vi "LVClass_Image get Fill Percent.vi"(0 "Image in":refnum<class "Image.lvclass">, 7 "Pixels to Average":u32, 11 "error in (no error)":errorcluster) -> (4 "Image out":refnum<class "Image.lvclass">, 6 "min":u32, 8 "max":u32, 10 "Fill Percent":sgl, 15 "error out":errorcluster)   [LabVIEW 2020, in "Image.lvclass"]
doc: "Image statistics computation.\n\n--------------------------------------------------------------------------------\n\n<B>ImageIn </B> : Image object.\n<B>ImageOut </B> : Image object.\n<B>nb_extreme_pixels </B> : Number of pixels to average for min or max computation.\n<B>min </B> : Average of the nb_extreme_pixels greatest elements.\n<B>max </B> : Average of the nb_extreme_pixels smallest elements.\n<B>fill_percentage </B> : Percentage of saturated pixels.\n<B>ErrorIn </B> : Error\n<B>ErrorOut </B> : Error\n\n--------------------------------------------------------------------------------"
uses:
  Image.lvclass
  Image.lvclass/Image.ctl
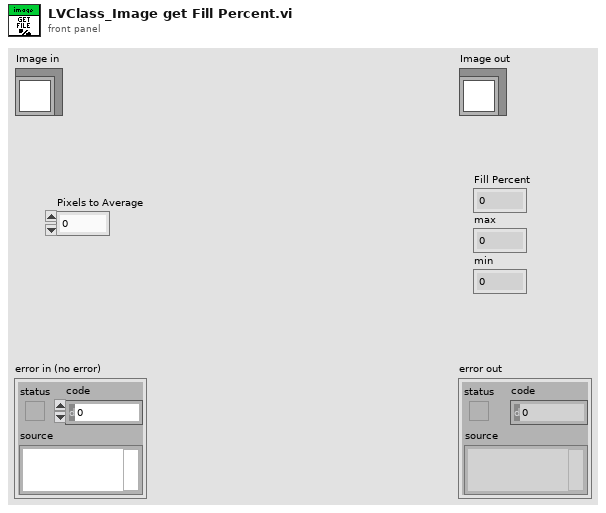
[diagram p1: front panel]
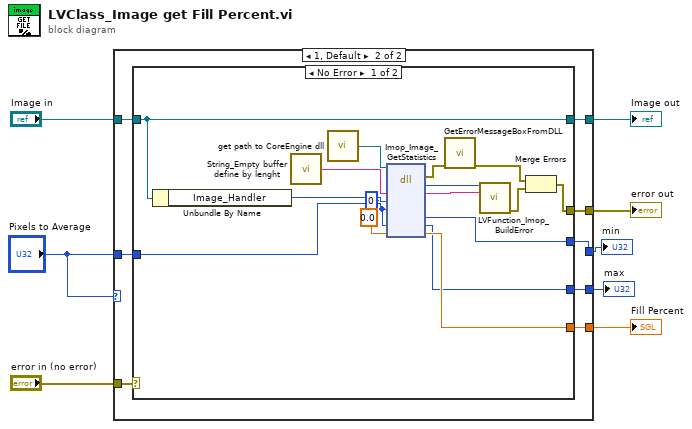
[diagram p0: block diagram]
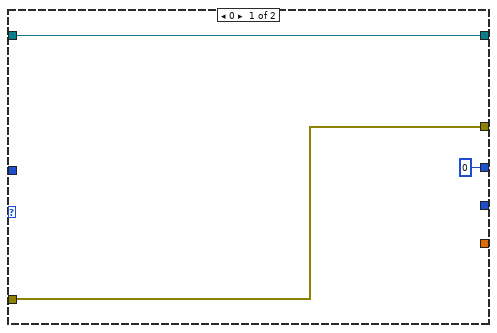
[diagram p2: hidden frame]
diagram:
  n1 = case shown="1, Default" "Pixels to Average" {
    tunnel: "error in (no error)" -> [w10 w19]
    tunnel: [w10 w18] -> w7
    tunnel: "Image in" -> [w11 w17]
    tunnel: [w11 w16] -> w5
    tunnel: [_ w15] -> w4
    tunnel: [u32 0 ("min") w14] -> w3
    tunnel: [_ w13] -> w2
    tunnel: "Pixels to Average" -> [_ w12]
    frame 0 {
    }
    frame 1, Default {
      n2 = case shown="No Error" w19 {
        selector: w19 -> [_ w37]
        tunnel: [w22 w37] -> w18
        tunnel: [w28 w36] -> w16
        tunnel: w17 -> [w28 w36]
        tunnel: [w29 _] -> w15
        tunnel: [w25 _] -> w14
        tunnel: [w24 _] -> w13
        tunnel: w12 -> [w20 _]
        frame No Error {
          n3 = Unbundle By Name(w28) -> ("Image_Handler"=w27:i32)
          n4 = call "String_Empty buffer define by lenght.vi"() -> ("Empty buffer"=w35:string)  [unwired: 1 in]
          n5 = call "get path to CoreEngine dll.vi"() -> ("path to c_interface_vc100.dll"=w32:path)  [unwired: 12 in, 3 out]
          n6 = dll-call lib="D:/soft/HASO_v3/SVN_trunk/ImOpCoreEngine4_LV2011/DLLs/c_interface_vc100.dll" fn="Imop_Image_GetStatistics"(path in=w32, "message"=w35, "Image compat"=w27, "Pixels to Average"=w20, "min"=u32 0, "max"=w20, "Fill_percent"=sgl 0.0 ("Fill Percent")) -> (error out=w31:errorcluster, "return type"=w34:i32, "message"=w33:string, "min"=w25:u32, "max"=w24:u32, "Fill_percent"=w29:sgl)  [unwired: 4 in, 1 out]
          n7 = call "GetErrorMessageBoxFromDLL.vi"("error IN"=w31) -> ("error OUT"=w21:errorcluster)  [unwired: 10 in]
          n8 = call "LVFunction_Imop_BuildError.vi"("code"=w34, "String to Prepend to source (\"\")"=w33) -> ("error out"=w23:errorcluster)  [unwired: 13 in]
          n9 = Merge Errors(w21, w23) -> (w22:errorcluster)
        }
        frame Error {
        }
      }
    }
  }
  "error out" <- w7
  "Image out" <- w5
  "Fill Percent" <- w4
  "min" <- w3
  "max" <- w2
